vi "calc_pixelhits.vi"(6 "error in":errorcluster, 9 "ImageAssemblerRK110612Spiral in":refnum<class "ImageAssemblerRK110612Spiral.lvclass">) -> (0 "error out":errorcluster, 3 "ImageAssemblerRK110612Spiral out":refnum<class "ImageAssemblerRK110612Spiral.lvclass">)   [LabVIEW 2010, in "ImageAssemblerRK110612Spiral.lvclass"]
uses:
  ImageAssemblerRK110612Spiral.lvclass
  ImageAssemblerRK110612Spiral.lvclass/ImageAssemblerRK110612Spiral.ctl
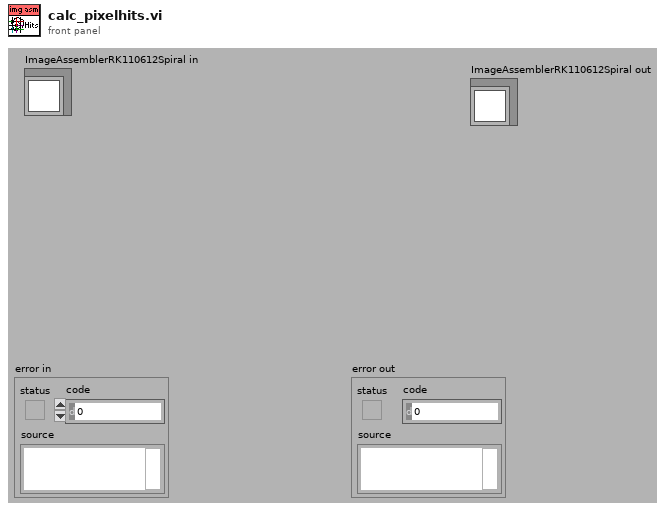
[diagram p1: front panel]
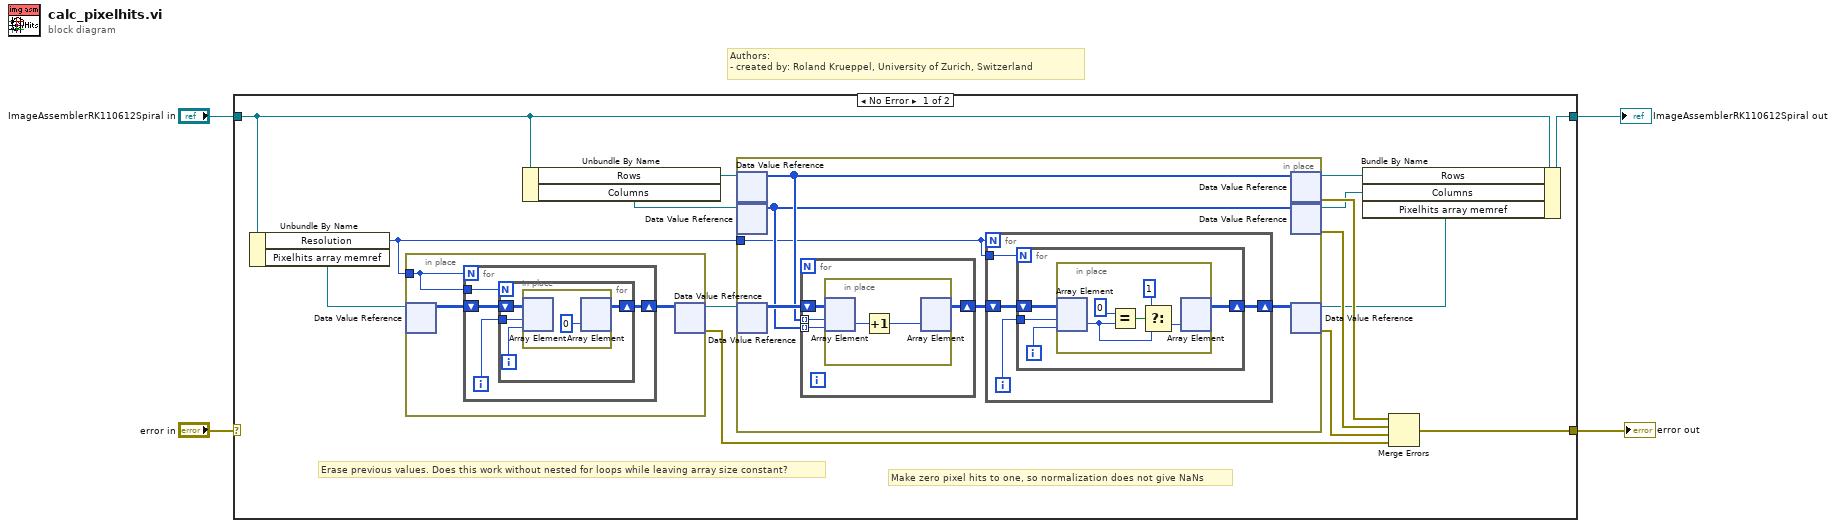
[diagram p0: block diagram]
diagram:
  # "Authors: \n- created by: Roland Krueppel, University of Zurich, Switzerland"
  n1 = case shown="No Error" "error in" {
    selector: "error in" -> [_ w58]
    tunnel: [w17 w58] -> w4
    tunnel: "ImageAssemblerRK110612Spiral in" -> [w9 w57]
    tunnel: [w5 w57] -> w1
    frame No Error {
      # "Erase previous values. Does this work without nested for loops while leaving array size constant?"
      # "Make zero pixel hits to one, so normalization does not give NaNs"
      n2 = Unbundle By Name(w9) -> ("Resolution"=w13:u16, "Pixelhits array memref"=w12:refnum<data-value>)
      n3 = in-place {
        in-place-border: w13 -> [w20]
        n4 = in-place-dvr #1(w12) -> (w22:u32[][])  [unwired: 1 out]
        n5 = for {
          N: w20 -> [_]
          tunnel: w20 -> [w26]
          shift-right: [w23] -> w21
          shift-left: w22 -> [w25]
          i -> [w24]
          n6 = for {
            N: w26 -> [_]
            shift-right: [w27] -> w23
            shift-left: w25 -> [w30]
            tunnel: w24 -> [w29]
            i -> [w28]
            n7 = in-place {
              n8 = in-place-array #2(w30, w29, w28) -> ()  [unwired: 1 out]
              n9 = in-place-array #2(u32 0 ("element")) -> (w27:u32[][])  [unwired: 2 out]
            }
          }
        }
        n10 = in-place-dvr #1(w21) -> (w19:refnum<data-value>, w16:errorcluster)
      }
      n11 = Unbundle By Name(w9) -> ("Rows"=w11:refnum<data-value>, "Columns"=w10:refnum<data-value>)
      n12 = in-place {
        in-place-border: w13 -> [w32]
        n13 = in-place-dvr #3(w11) -> (w34:i32[])  [unwired: 1 out]
        n14 = in-place-dvr #4(w10) -> (w33:i32[])  [unwired: 1 out]
        n15 = in-place-dvr #5(w19) -> (w35:u32[][])  [unwired: 1 out]
        n16 = for {
          shift-right: [w53] -> w37
          shift-left: w35 -> [w54]
          tunnel: w34 -> [w52] mode=indexing
          tunnel: w33 -> [w51] mode=indexing
          n17 = in-place {
            n18 = in-place-array #6(w54, w52, w51) -> (w56:u32)
            n19 = Increment(x=w56) -> (x+1=w55:u32)
            n20 = in-place-array #6(w55) -> (w53:u32[][])  [unwired: 2 out]
          }
        }
        n21 = for {
          N: w32 -> [_]
          shift-right: [w40] -> w36
          shift-left: w37 -> [w41]
          tunnel: w32 -> [w39]
          i -> [w38]
          n22 = for {
            N: w39 -> [_]
            shift-right: [w42] -> w40
            shift-left: w41 -> [w45]
            tunnel: w38 -> [w44]
            i -> [w43]
            n23 = in-place {
              n24 = in-place-array #7(w45, w44, w43) -> (w46:u32)
              n25 = Equal?(x=u32 0, y=w46) -> (x = y?=w50:bool)
              n26 = Select(t=u32 1, s=w50, f=w46) -> (s? t:f=w47:u32)
              n27 = in-place-array #7(w47) -> (w42:u32[][])  [unwired: 2 out]
            }
          }
        }
        n28 = in-place-dvr #3(w34) -> (w8:refnum<data-value>, w14:errorcluster)
        n29 = in-place-dvr #4(w33) -> (w7:refnum<data-value>, w15:errorcluster)
        n30 = in-place-dvr #5(w36) -> (w6:refnum<data-value>, w18:errorcluster)
      }
      n31 = Bundle By Name(cluster=w9, "Rows"=w8, "Columns"=w7, "Pixelhits array memref"=w6) -> (w5:refnum<class "ImageAssemblerRK110612Spiral.lvclass">)
      n32 = Merge Errors(w14, w15, w18, w16) -> (w17:errorcluster)
    }
    frame Error {
    }
  }
  "error out" <- w4
  "ImageAssemblerRK110612Spiral out" <- w1
